vi "AktuelleTDMS.vi"(0 "AktuelleTDMS":refnum<k34>, 1 "error in TDMSopen":errorcluster, 2 "Dateiordner":path, 5 "NächsteTDMS":refnum<k34>, 7 "NeuerZyklus?":bool, 9 "Methodennummer":i32, 11 "Zyklnumges":i32, 12 "error in TDMSclose":errorcluster, 13 "Dateiname":string) -> (4 "AktuelleTDMS":refnum<k34>, 6 "error out TDMSopen":errorcluster, 10 "error out TDMSclose":errorcluster, 15 "NächsteTDMS":refnum<k34>)   [LabVIEW 2010]
uses:
  <vilib>/addons/internet/NI_InternetTK_FTP_VIs.lvlib
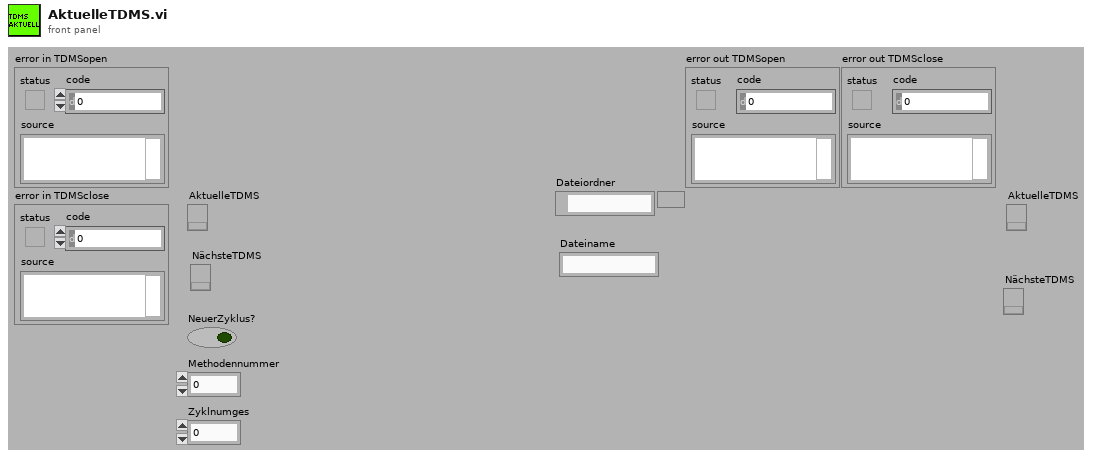
[diagram p1: front panel]
types:
  T1 = enum16{"open", "open or create", "create or replace", "create", "open (read-only)"}
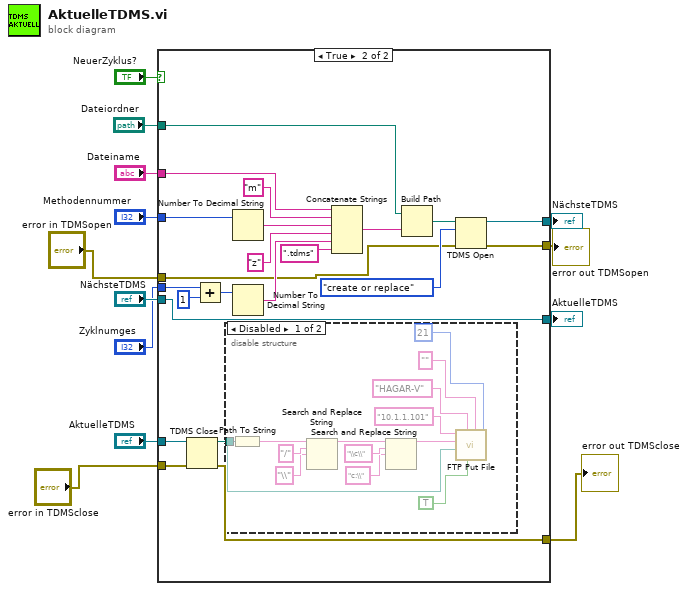
[diagram p0: block diagram]
diagram:
  n1 = case shown="True" "NeuerZyklus?" {
    tunnel: "Zyklnumges" -> [_ w38]
    tunnel: "AktuelleTDMS" -> [w17 w23]
    tunnel: "NächsteTDMS" -> [w16 w39]
    tunnel: [w17 w39] -> w13
    tunnel: [w16 w37] -> w9
    tunnel: "Dateiname" -> [_ w36]
    tunnel: "Dateiordner" -> [_ w35]
    tunnel: "Methodennummer" -> [_ w34]
    tunnel: "error in TDMSopen" -> [w15 w21]
    tunnel: [w15 w20] -> w3
    tunnel: "error in TDMSclose" -> [w14 w19]
    tunnel: [w14 w18] -> w1
    frame False {
    }
    frame True {
      n2 = TDMS Close(8:w19, 11:w23) -> (0:w18:errorcluster, 3:w22:path)
      n3 = Add(x=w38, y=1) -> (x+y=w31:i32)
      n4 = disable-structure shown="Disabled" {
        disable-tunnel: w22 -> [w47 _]
        frame Disabled {
          n5 = Path To String(path=w47) -> (string=w46:string)
          n6 = Search and Replace String(input string=w46, search string="/", replace string="\\" ("replace string (\"\")")) -> (result string=w43:string)  [unwired: 5 in, 3 out]
          n7 = Search and Replace String(input string=w43, search string="\\c\\", replace string="c:\\" ("replace string (\"\")")) -> (result string=w40:string)  [unwired: 5 in, 3 out]
          n8 = call <vilib>:"FTP Put File.vi"("remote port (21)"=u16 21, "password"="" ("user"), "binary (F)"=TRUE, "user"="HAGAR-V", "local path"=w47, "remote path"=w40, "host"="10.1.1.101") -> ()  [unwired: 3 in, 2 out]
        }
        frame Enabled {
        }
      }
      n9 = Number To Decimal String(number=w34) -> (decimal integer string=w26:string)  [unwired: 1 in]
      n10 = Number To Decimal String(number=w31) -> (decimal integer string=w24:string)  [unwired: 1 in]
      n11 = Concatenate Strings(w36, "m", w26, "z", w24, ".tdms" ("String")) -> (w30:string)
      n12 = Build Path(base path=w35, name or relative path=w30) -> (appended path=w32:path)
      n13 = TDMS Open(8:w21, 10:T1."create or replace" ("Operation (0:Öffnen)"), 11:w32) -> (0:w20:errorcluster, 3:w37:refnum<k34>)  [unwired: 3 in]
    }
  }
  "AktuelleTDMS" <- w13
  "NächsteTDMS" <- w9
  "error out TDMSopen" <- w3
  "error out TDMSclose" <- w1
